vi "RTS Write Point File.vi"(8 "Error In":errorcluster, 9 "Header Save Array Input":T1[](array[typedef]), 10 "Point Data":T2[](array[typedef]), 11 "Path":path) -> (0 "Error Out":errorcluster)   [LabVIEW 2018]
uses:
  Type Definitions/RTS Point File.ctl
  Washer DOE/Type Definitions/DOE Data Save Modifier.ctl
panel:
  out "Save Data":string
  in  "Debug":T2[](array[typedef])=[{"Title"="FA MID", "Name"="TC1", "Point"=1, "Plot"=TRUE, "Trend"=TRUE, "Cycle"=TRUE, "Field"=0, "Row On (Save Data)"=TRUE, "Group"=1}, {"Title"="FF MID", "Name"="TC2", "Point"=2, "Plot"=TRUE, "Trend"=TRUE, "Cycle"=TRUE, "Field"=1, "Row On (Save Data)"=FALSE, "Group"=2}, {"Title"="FA3", "Name"="TC3", "Point"=3, "Plot"=TRUE, "Trend"=TRUE, "Cycle"=TRUE, "Field"=2, "Row On (Save Data)"=FALSE, "Group"=1}, {"Title"="FC THERMISTER", "Name"="TC4", "Point"=4, "Plot"=TRUE, "Trend"=TRUE, "Cycle"=TRUE, "Field"=3, "Row On (Save Data)"=FALSE, "Group"=1}, {"Title"="FC SUPPLY", "Name"="TC5", "Point"=5, "Plot"=TRUE, "Trend"=TRUE, "Cycle"=TRUE, "Field"=4, "Row On (Save Data)"=FALSE, "Group"=1}, {"Title"="RC THERM WATERBOX", "Name"="TC6", "Point"=6, "Plot"=TRUE, "Trend"=TRUE, "Cycle"=TRUE, "Field"=5, "Row On (Save Data)"=FALSE, "Group"=1}, {"Title"="RC DIFF BOT RT", "Name"="TC7", "Point"=7, "Plot"=TRUE, "Trend"=TRUE, "Cycle"=TRUE, "Field"=6, "Row On (Save Data)"=FALSE, "Group"=1}, {"Title"="RC SUPPLY", "Name"="TC8", "Point"=8, "Plot"=TRUE, "Trend"=TRUE, "Cycle"=TRUE, "Field"=7, "Row On (Save Data)"=FALSE, "Group"=1}, {"Title"="CU URR", "Name"="TC9", "Point"=9, "Plot"=TRUE, "Trend"=TRUE, "Cycle"=TRUE, "Field"=8, "Row On (Save Data)"=FALSE, "Group"=1}, {"Title"="CU LLF", "Name"="TC10", "Point"=10, "Plot"=TRUE, "Trend"=TRUE, "Cycle"=TRUE, "Field"=9, "Row On (Save Data)"=FALSE, "Group"=1}, {"Title"="FF MID", "Name"="TC11", "Point"=11, "Plot"=TRUE, "Trend"=TRUE, "Cycle"=TRUE, "Field"=10, "Row On (Save Data)"=TRUE, "Group"=2}, {"Title"="FF2", "Name"="TC12", "Point"=12, "Plot"=TRUE, "Trend"=TRUE, "Cycle"=TRUE, "Field"=11, "Row On (Save Data)"=FALSE, "Group"=2}, {"Title"="FF3", "Name"="TC13", "Point"=13, "Plot"=TRUE, "Trend"=TRUE, "Cycle"=TRUE, "Field"=12, "Row On (Save Data)"=FALSE, "Group"=2}, {"Title"="RC R-SIDE WALL", "Name"="TC14", "Point"=14, "Plot"=TRUE, "Trend"=TRUE, "Cycle"=TRUE, "Field"=13, "Row On (Save Data)"=FALSE, "Group"=2}, {"Title"="EVAPIN", "Name"="TC15", "Point"=15, "Plot"=TRUE, "Trend"=TRUE, "Cycle"=TRUE, "Field"=14, "Row On (Save Data)"=FALSE, "Group"=2}, {"Title"="EVAPOUT", "Name"="TC16", "Point"=16, "Plot"=TRUE, "Trend"=TRUE, "Cycle"=TRUE, "Field"=15, "Row On (Save Data)"=FALSE, "Group"=2}, {"Title"="SUCT6\"COMP", "Name"="TC17", "Point"=17, "Plot"=TRUE, "Trend"=TRUE, "Cycle"=TRUE, "Field"=16, "Row On (Save Data)"=FALSE, "Group"=2}, {"Title"="DOME", "Name"="TC18", "Point"=18, "Plot"=TRUE, "Trend"=TRUE, "Cycle"=TRUE, "Field"=17, "Row On (Save Data)"=FALSE, "Group"=2}, {"Title"="1STDISCH", "Name"="TC19", "Point"=19, "Plot"=TRUE, "Trend"=TRUE, "Cycle"=TRUE, "Field"=18, "Row On (Save Data)"=FALSE, "Group"=2}, {"Title"="CONDMID", "Name"="TC20", "Point"=20, "Plot"=TRUE, "Trend"=TRUE, "Cycle"=TRUE, "Field"=19, "Row On (Save Data)"=FALSE, "Group"=2}, {"Title"="HLIN", "Name"="TC21", "Point"=21, "Plot"=TRUE, "Trend"=TRUE, "Cycle"=TRUE, "Field"=20, "Row On (Save Data)"=FALSE, "Group"=2}, {"Title"="HLOUT", "Name"="TC22", "Point"=22, "Plot"=TRUE, "Trend"=TRUE, "Cycle"=TRUE, "Field"=21, "Row On (Save Data)"=FALSE, "Group"=2}, {"Title"="AMBLEFTBOT", "Name"="AMBLEFTBOT", "Point"=23, "Plot"=TRUE, "Trend"=TRUE, "Cycle"=TRUE, "Field"=22, "Row On (Save Data)"=TRUE, "Group"=2}, {"Title"="AMBLEFT", "Name"="AMBLEFT", "Point"=24, "Plot"=TRUE, "Trend"=TRUE, "Cycle"=TRUE, "Field"=23, "Row On (Save Data)"=TRUE, "Group"=3}, {"Title"="AMBLEFTTOP", "Name"="AMBLEFTTOP", "Point"=25, "Plot"=TRUE, "Trend"=TRUE, "Cycle"=TRUE, "Field"=24, "Row On (Save Data)"=TRUE, "Group"=3}, {"Title"="AMBRIGHTBOT", "Name"="AMBRIGHTBOT", "Point"=26, "Plot"=TRUE, "Trend"=TRUE, "Cycle"=TRUE, "Field"=25, "Row On (Save Data)"=TRUE, "Group"=3}, {"Title"="AMBRIGHT", "Name"="AMBRIGHT", "Point"=27, "Plot"=TRUE, "Trend"=TRUE, "Cycle"=TRUE, "Field"=26, "Row On (Save Data)"=TRUE, "Group"=3}, {"Title"="AMBRIGHTTOP", "Name"="AMBRIGHTTOP", "Point"=28, "Plot"=TRUE, "Trend"=TRUE, "Cycle"=TRUE, "Field"=27, "Row On (Save Data)"=TRUE, "Group"=3}]
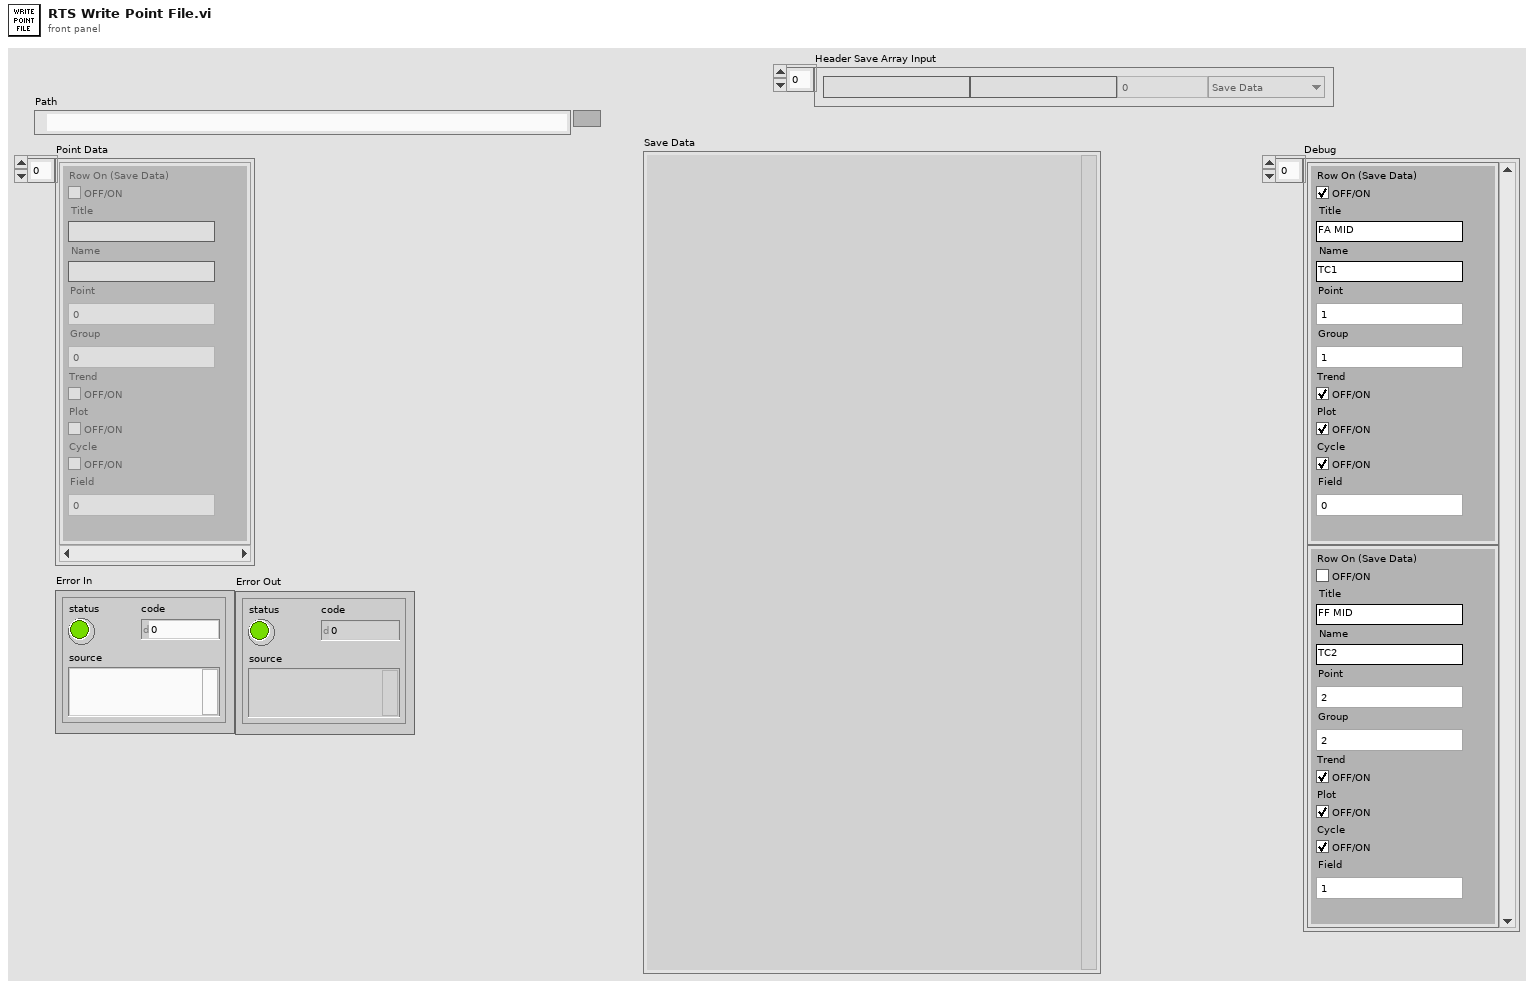
[diagram p1: front panel]
types:
  T1 = typedef "DOE Data Save Modifier.ctl" = cluster{"Name":string, "Title":string, "Save Status":enum16{"Save Data", "Don't Save Data"}, "Group":u8, "Field":u8}
  T2 = typedef "RTS Point File.ctl" = cluster{"Title":string, "Name":string, "Point":u8, "Plot":bool, "Trend":bool, "Cycle":bool, "Field":u8, "Row On (Save Data)":bool, "Group":u8}
  T3 = enum16{"open", "replace", "create", "open or create", "replace or create", "replace or create with confirmation"}
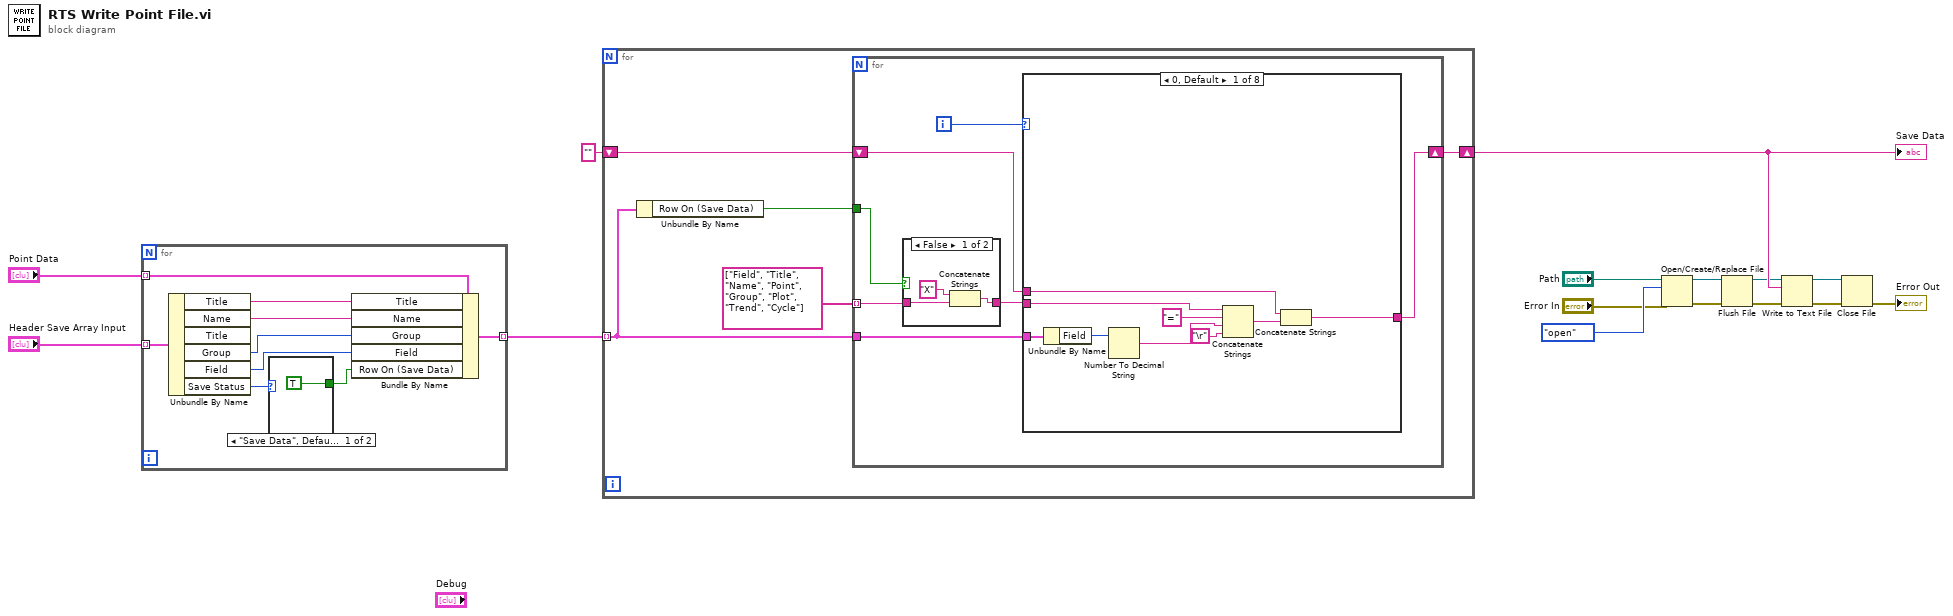
[diagram p0: block diagram]
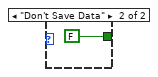
[diagram p2: hidden frame]
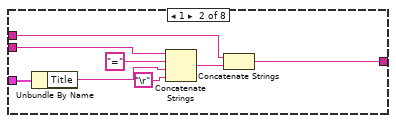
[diagram p3: hidden frame]
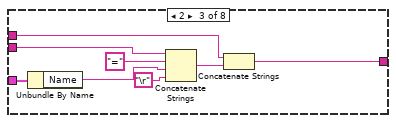
[diagram p4: hidden frame]
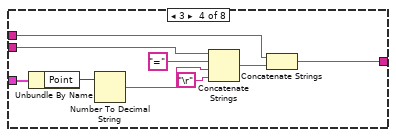
[diagram p5: hidden frame]
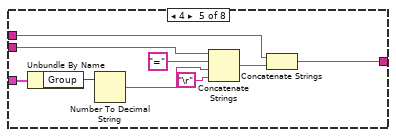
[diagram p6: hidden frame]
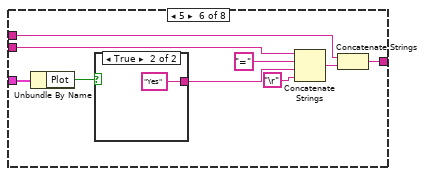
[diagram p7: hidden frame]
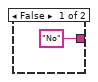
[diagram p8: hidden frame]
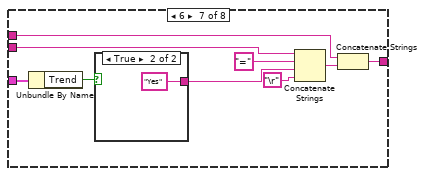
[diagram p9: hidden frame]
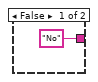
[diagram p10: hidden frame]
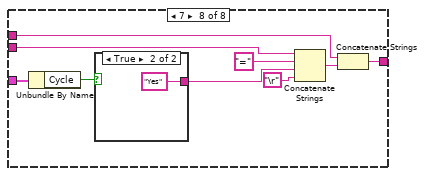
[diagram p11: hidden frame]
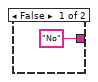
[diagram p12: hidden frame]
diagram:
  n1 = for {
    tunnel: "Point Data" -> [w24] mode=indexing
    tunnel: [w23] -> w6 mode=indexing
    tunnel: "Header Save Array Input" -> [w22] mode=indexing
    n2 = Unbundle By Name(w22) -> ("Title"=w21:string, "Name"=w20:string, "Group"=w19:u8, "Field"=w18:u8, "Save Status"=w17:enum16{"Save Data", "Don't Save Data"})  [unwired: 1 out]
    n3 = case shown="\"Save Data\", Default" w17 {
      tunnel: [TRUE FALSE] -> w16
      frame "Save Data", Default {
      }
      frame "Don't Save Data" {
      }
    }
    n4 = Bundle By Name(cluster=w24, "Title"=w21, "Name"=w20, "Group"=w19, "Field"=w18, "Row On (Save Data)"=w16) -> (w23:T2)
  }
  n5 = for {
    tunnel: w6 -> [w29] mode=indexing
    shift-right: [w28] -> w12
    shift-left: "" -> [w27]
    n6 = Unbundle By Name(w29) -> ("Row On (Save Data)"=w30:bool)
    n7 = for {
      tunnel: string[] ["Field", "Title", "Name", "Point", "Group", "Plot", "Trend", "Cycle"] ("subarray 2") -> [w33] mode=indexing
      tunnel: w30 -> [w34]
      tunnel: w29 -> [w37]
      shift-right: [w35] -> w28
      shift-left: w27 -> [w36]
      i -> [w38]
      n8 = case shown="False" w34 {
        tunnel: [w117 w118] -> w32
        tunnel: w33 -> [w116 w118]
        frame False {
          n9 = Concatenate Strings("X" ("string"), w116) -> (w117:string)
        }
        frame True {
        }
      }
      n10 = case shown="0, Default" w38 {
        tunnel: w37 -> [w47 w55 w63 w72 w81 w90 w101 w112]
        tunnel: w32 -> [w46 w53 w60 w64 w73 w82 w93 w104]
        tunnel: w36 -> [w41 w50 w58 w67 w76 w84 w94 w105]
        tunnel: [w40 w48 w56 w65 w74 w83 w95 w106] -> w35
        frame 0, Default {
          n11 = Unbundle By Name(w47) -> ("Field"=w44:u8)
          n12 = Number To Decimal String(number=w44) -> (decimal integer string=w43:string)  [unwired: 1 in]
          n13 = Concatenate Strings(w46, "=" ("string"), w43, "\r") -> (w42:string)
          n14 = Concatenate Strings(w41, w42) -> (w40:string)
        }
        frame 1 {
          n15 = Unbundle By Name(w55) -> ("Title"=w51:string)
          n16 = Concatenate Strings(w53, "=" ("string"), w51, "\r") -> (w49:string)
          n17 = Concatenate Strings(w50, w49) -> (w48:string)
        }
        frame 2 {
          n18 = Unbundle By Name(w63) -> ("Name"=w59:string)
          n19 = Concatenate Strings(w60, "=" ("string"), w59, "\r") -> (w57:string)
          n20 = Concatenate Strings(w58, w57) -> (w56:string)
        }
        frame 3 {
          n21 = Unbundle By Name(w72) -> ("Point"=w66:u8)
          n22 = Number To Decimal String(number=w66) -> (decimal integer string=w70:string)  [unwired: 1 in]
          n23 = Concatenate Strings(w64, "=" ("string"), w70, "\r") -> (w69:string)
          n24 = Concatenate Strings(w67, w69) -> (w65:string)
        }
        frame 4 {
          n25 = Unbundle By Name(w81) -> ("Group"=w75:u8)
          n26 = Number To Decimal String(number=w75) -> (decimal integer string=w79:string)  [unwired: 1 in]
          n27 = Concatenate Strings(w73, "=" ("string"), w79, "\r") -> (w78:string)
          n28 = Concatenate Strings(w76, w78) -> (w74:string)
        }
        frame 5 {
          n29 = Unbundle By Name(w90) -> ("Plot"=w89:bool)
          n30 = case shown="True" w89 {
            tunnel: ["No" "Yes"] -> w86
            frame False {
            }
            frame True {
            }
          }
          n31 = Concatenate Strings(w82, "=" ("string"), w86, "\r") -> (w85:string)
          n32 = Concatenate Strings(w84, w85) -> (w83:string)
        }
        frame 6 {
          n33 = Unbundle By Name(w101) -> ("Trend"=w97:bool)
          n34 = case shown="True" w97 {
            tunnel: ["No" "Yes"] -> w98
            frame False {
            }
            frame True {
            }
          }
          n35 = Concatenate Strings(w93, "=" ("string"), w98, "\r") -> (w96:string)
          n36 = Concatenate Strings(w94, w96) -> (w95:string)
        }
        frame 7 {
          n37 = Unbundle By Name(w112) -> ("Cycle"=w108:bool)
          n38 = case shown="True" w108 {
            tunnel: ["No" "Yes"] -> w109
            frame False {
            }
            frame True {
            }
          }
          n39 = Concatenate Strings(w104, "=" ("string"), w109, "\r") -> (w107:string)
          n40 = Concatenate Strings(w105, w107) -> (w106:string)
        }
      }
    }
  }
  "Save Data" <- w12
  n41 = Open/Create/Replace File(file path (use dialog)="Path", error in="Error In", operation (0:open)=T3."open") -> (refnum out=w4:refnum<file>, error out=w3:errorcluster)  [unwired: 3 in, 1 out]
  n42 = Flush File(refnum=w4, error in=w3) -> (refnum out=w2:refnum<file>, error out=w1:errorcluster)
  n43 = Write to Text File(file (use dialog)=w2, text=w12, error in=w1) -> (refnum out=w10:refnum<file>, error out=w11:errorcluster)  [unwired: 1 in, 1 out]
  n44 = Close File(refnum=w10, error in=w11) -> (error out=→"Error Out":errorcluster)  [unwired: 1 out]
